vi "DataHandler Type.vi"(8 "error in (no error)":errorcluster, 11 "RedlinesDataHandler in":refnum<class "RedlinesDataHandler.lvclass">) -> (0 "error out":errorcluster, 2 "DataHandler Type":string, 3 "RedlinesDataHandler out":refnum<class "RedlinesDataHandler.lvclass">)   [LabVIEW 2020, in "VolatusDataProcessing.lvlib" / "RedlinesDataHandler.lvclass"]
uses:
  RedlinesDataHandler.lvclass
  RedlinesDataHandler.lvclass/RedlinesDataHandler.ctl
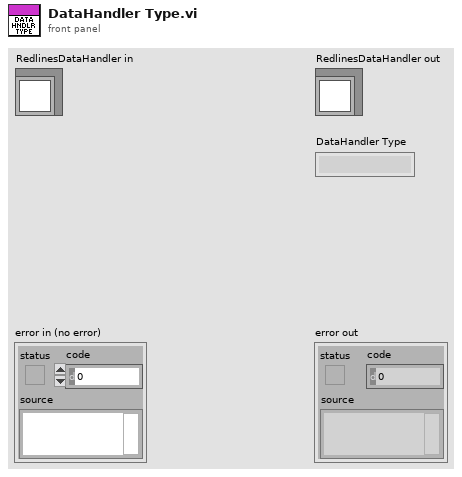
[diagram p1: front panel]
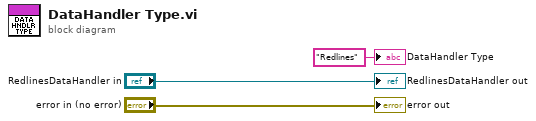
[diagram p0: block diagram]
diagram:
  "error out" <- "error in (no error)"
  "RedlinesDataHandler out" <- "RedlinesDataHandler in"
  "DataHandler Type" <- "Redlines" ("DataHandler Type")
